vi "SPO2 (SubVI).vi"(4 "I_max_lam1":dbl, 5 "eps_Hb_lam2":dbl, 6 "I_min_lam2":dbl, 7 "eps_Hb_lam1":dbl, 8 "I_max_lam2":dbl, 9 "eps_HbO2_lam2":dbl, 10 "I_min_lam1":dbl, 11 "eps_HbO2_lam1":dbl) -> (3 "Numeric":dbl)   [LabVIEW 2021]
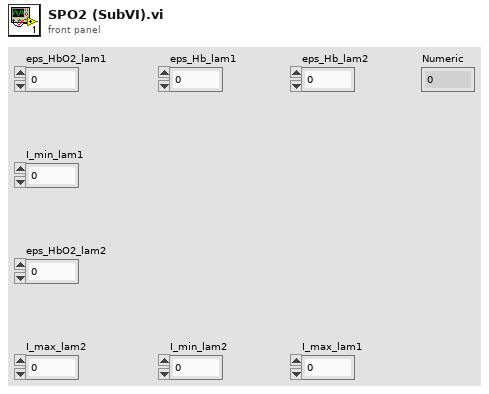
[diagram p1: front panel]
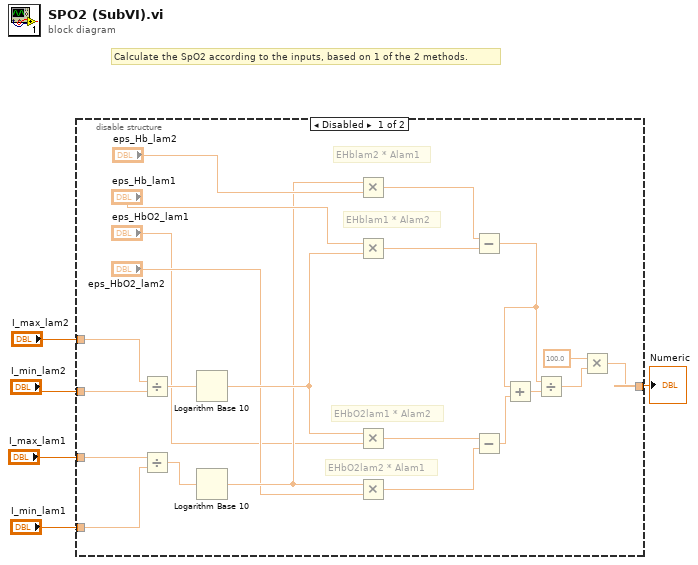
[diagram p0: block diagram]
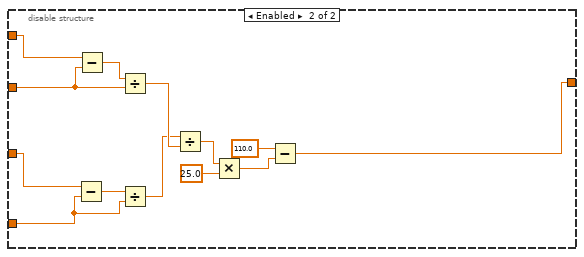
[diagram p2: hidden frame]
diagram:
  # "Calculate the SpO2 according to the inputs, based on 1 of the 2 methods."
  n1 = disable-structure shown="Disabled" {
    disable-tunnel: [w7 w28] -> w5
    disable-tunnel: "I_min_lam2" -> [w13 w37]
    disable-tunnel: "I_max_lam2" -> [w12 w40]
    disable-tunnel: "I_min_lam1" -> [w11 w35]
    disable-tunnel: "I_max_lam1" -> [w10 w39]
    frame Disabled {
      # "EHbO2lam2 * Alam1"
      # "EHbO2lam1 * Alam2"
      # "EHblam1 * Alam2"
      # "EHblam2 * Alam1"
      n2 = Divide(x=w12, y=w13) -> (x/y=w24:dbl)
      n3 = Divide(x=w10, y=w11) -> (x/y=w22:dbl)
      n4 = Logarithm Base 10(1:w24) -> (0:w25:dbl)
      n5 = Logarithm Base 10(1:w22) -> (0:w23:dbl)
      n6 = Multiply(x=w23, y="eps_Hb_lam2") -> (x*y=w14:dbl)
      n7 = Multiply(x="eps_Hb_lam1", y=w25) -> (x*y=w15:dbl)
      n8 = Multiply(x=w25, y="eps_HbO2_lam1") -> (x*y=w18:dbl)
      n9 = Multiply(x=w23, y="eps_HbO2_lam2") -> (x*y=w19:dbl)
      n10 = Subtract(x=w14, y=w15) -> (x-y=w9:dbl)
      n11 = Subtract(x=w18, y=w19) -> (x-y=w20:dbl)
      n12 = Add(x=w9, y=w20) -> (x+y=w21:dbl)
      n13 = Divide(x=w9, y=w21) -> (x/y=w8:dbl)
      n14 = Multiply(x=100.0, y=w8) -> (x*y=w7:dbl)
    }
    frame Enabled {
      n15 = Subtract(x=w39, y=w35) -> (x-y=w36:dbl)
      n16 = Subtract(x=w40, y=w37) -> (x-y=w38:dbl)
      n17 = Divide(x=w38, y=w37) -> (x/y=w34:dbl)
      n18 = Divide(x=w36, y=w35) -> (x/y=w33:dbl)
      n19 = Divide(x=w33, y=w34) -> (x/y=w32:dbl)
      n20 = Multiply(x=w32, y=25.0) -> (x*y=w30:dbl)
      n21 = Subtract(x=110.0, y=w30) -> (x-y=w28:dbl)
    }
  }
  "Numeric" <- w5
